vi "SLSC Get Channels to Remove.vi"(7 "Channels Created":string[](array[string]), 10 "All Channel Values":dbl[](array[numeric]), 11 "All Channels":string[](array[string])) -> (1 "Channels to be Deleted":string[](array[string]), 2 "Channel Values":dbl[](array[numeric]), 3 "Channels to be Added":string[](array[string]))   [LabVIEW 2015, in "SLSC EDS System Explorer.lvlib"]
uses:
  System Explorer/SLSC EDS System Explorer.lvlib
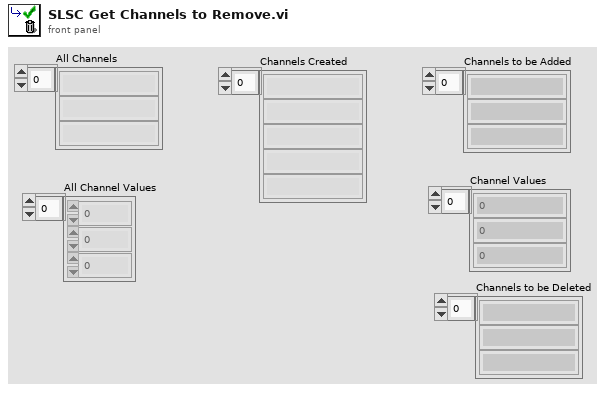
[diagram p1: front panel]
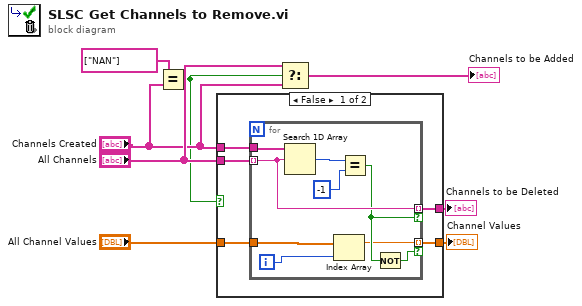
[diagram p0: block diagram]
diagram:
  n1 = Equal?(x=string[] ["NAN"] ("TreeItem Channels"), y="Channels Created") -> (x = y?=w1:bool)
  n2 = case shown="False" w1 {
    tunnel: "All Channel Values" -> [w13 w23]
    tunnel: [w12 w23] -> w7
    tunnel: [w11 _] -> w6
    tunnel: "All Channels" -> [w10 _]
    tunnel: "Channels Created" -> [w9 _]
    frame False {
      n3 = for {
        tunnel: w10 -> [w18] mode=indexing
        tunnel: w13 -> [w19]
        tunnel: w9 -> [w22]
        tunnel: [w15] -> w12 mode=indexing if=w17
        tunnel: [w18] -> w11 mode=indexing if=w16
        i -> [w14]
        n4 = Search 1D Array(1D array=w22, element=w18) -> (index of element=w21:i32)  [unwired: 1 in]
        n5 = Index Array(array=w19, index=w14) -> (element=w15:dbl)
        n6 = Equal?(x=w21, y=-1) -> (x = y?=w16:bool)
        n7 = Not(x=w16) -> (.not. x?=w17:bool)
      }
    }
    frame True {
    }
  }
  "Channels to be Deleted" <- w6
  "Channel Values" <- w7
  n8 = Select(t="All Channels", s=w1, f="Channels Created") -> (s? t:f=→"Channels to be Added":string[])
